vi "Voltage - Finite Output.vi"() -> ()   [LabVIEW 2011]
doc: "This example demonstrates how to generate a finite amount of data from a buffer in your computer's memory."
uses:
  <libdir>/resource/objmgr/daqmx.rc
  <vilib>/DAQmx/create/channels.llb/DAQmx Create Channel (AO-Voltage-Basic).vi
  <vilib>/DAQmx/configure/trigger.llb/DAQmx Start Trigger (Analog Edge).vi
  <vilib>/DAQmx/configure/trigger.llb/DAQmx Start Trigger (Digital Edge).vi
  <vilib>/Utility/error.llb/DialogType.ctl
  <vilib>/DAQmx/write.llb/DAQmx Write (Analog Wfm 1Chan NSamp).vi
  <vilib>/DAQmx/configure/timing.llb/DAQmx Timing (Use Waveform).vi
  <vilib>/Utility/file.llb/Read Delimited Spreadsheet (DBL).vi
panel:
  out "Samples":i32
  out "appended path":path
  in  "amplitude":dbl=1.0 format="%0.2p"
  in  "Trigger Type":T1(tab)
  in  "Edge":i32(ring)=10280 items=["Rising"=10280, "Falling"=10171]
  in  "Digital Trigger Source":tag
  in  "Level (V)":dbl format="%0.2f"
  in  "Hysteresis (V)":dbl
  in  "Slope":i32(ring)=10280 items=["Rising"=10280, "Falling"=10171]
  in  "Analog Trigger Source":string="APFI0"
  out "Waveform Graph":waveform(dbl)(graph)
  in  "Sample Rate":dbl=1000.0
  in  "Physical Channel(s)":tag="Dev1/ao0"
  out "Actual Sample Rate":dbl=1000.0 format="%0.2f"
  # "Channel Settings"
  # "Output"
  # "Timing and Buffer Settings"
  # "Trigger Settings"
  # "Waveform Settings"
  # "The number of elements in the waveform array must equal the number of channels in the task."
  # "To configure and use a start trigger you must have the necessary tab selected above.  Not all hardware supports triggering--refer to your device documentation for more info."
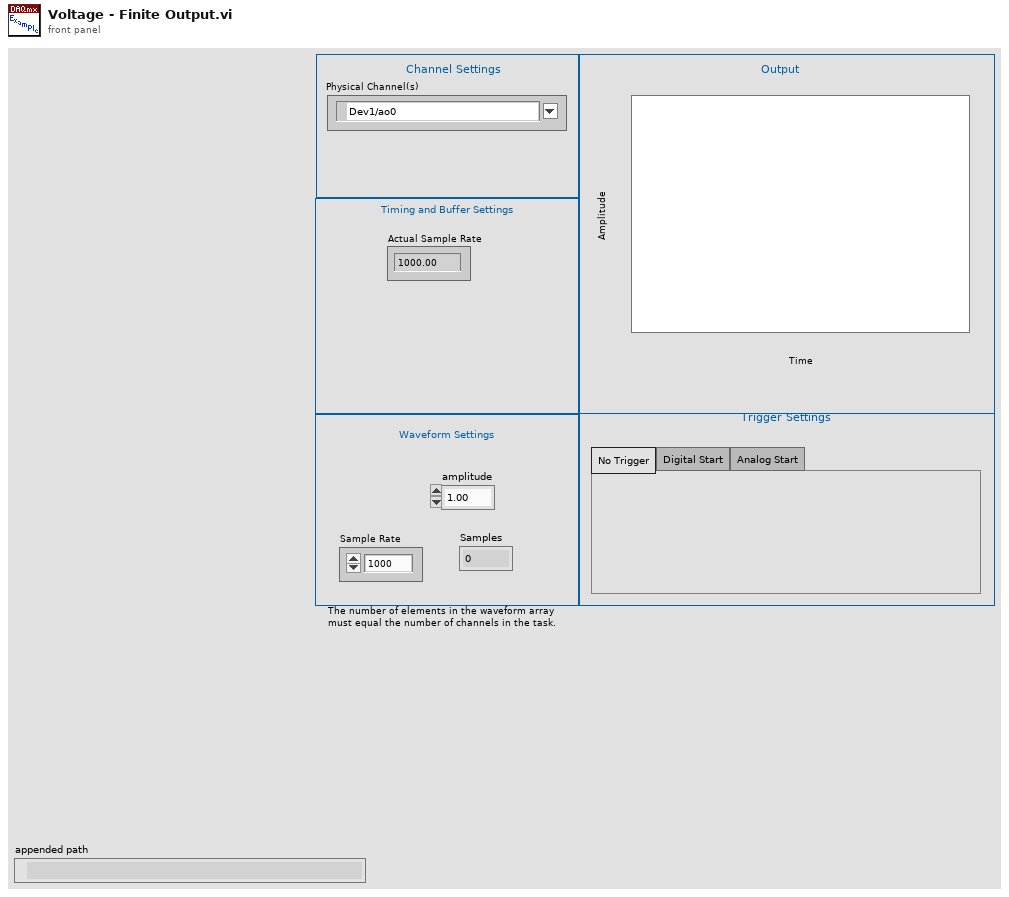
[diagram p1: front panel]
types:
  T1 = enum32{"No Trigger", "Digital Start", "Analog Start"}
  T2 = typedef "DialogType.ctl" = u16
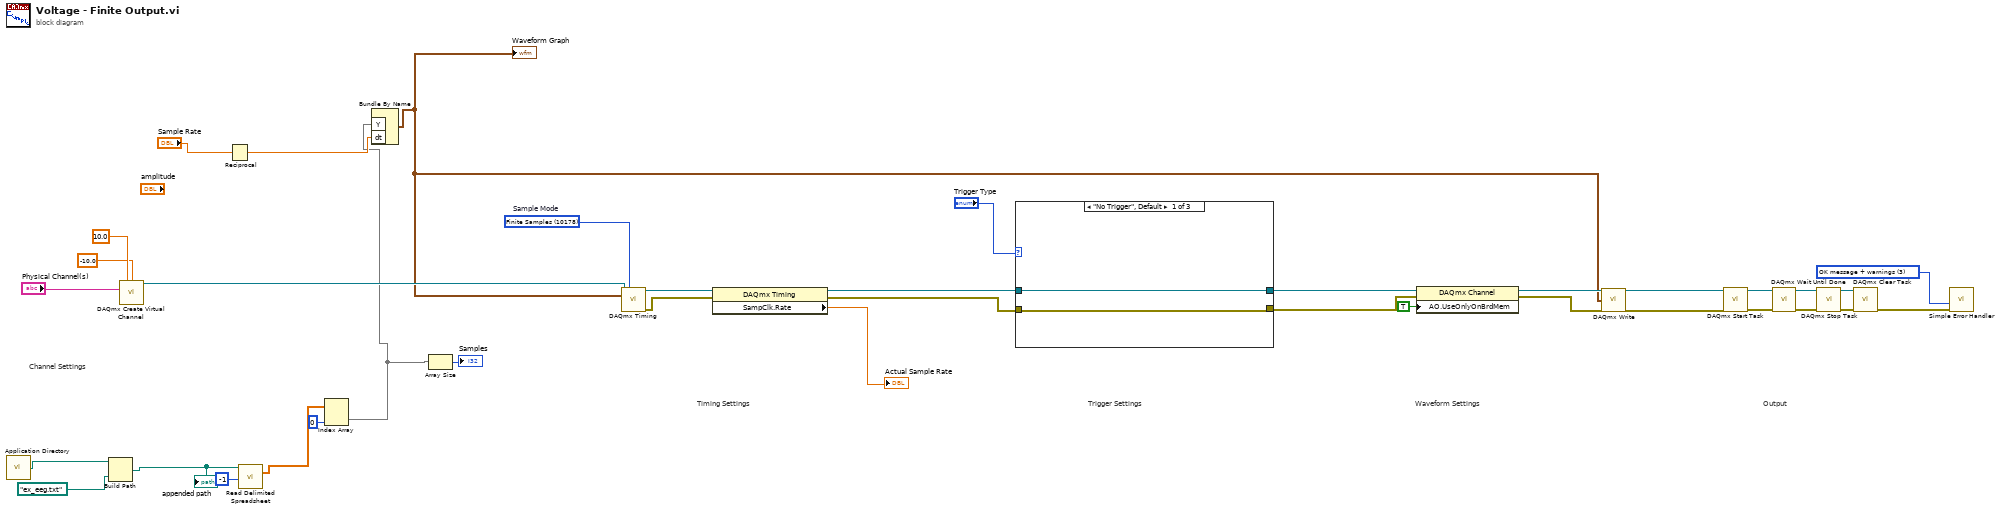
[diagram p0: block diagram]
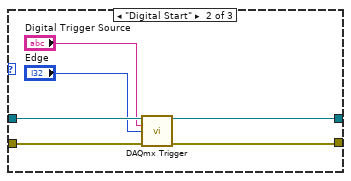
[diagram p2: hidden frame]
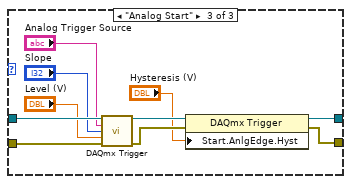
[diagram p3: hidden frame]
diagram:
  w19 = T2 3 items=["no dialog", "OK message", "continue or stop message", "OK message + warnings", "continue/stop + warnings"] ("type of dialog (OK msg:1)")
  w35 = 10178 items=["Finite Samples"=10178, "Continuous Samples"=10123, "Hardware Timed Single Point"=12522]  # Sample Mode
  # "Output"
  # "Trigger Settings"
  # "Waveform Settings"
  # "Timing Settings"
  # "Channel Settings"
  n1 = call <vilib>:"Application Directory.vi"() -> ("Application Directory"=w7:path)
  n2 = Build Path(base path=w7, name or relative path=path "ex_eeg.txt" ("file path (dialog if empty)")) -> (appended path=w8:path)
  "appended path" <- w8
  n3 = call-poly <vilib>:"DAQmx Create Virtual Channel.vi"("maximum value"=10.0, "minimum value"=-10.0, "physical channels"="Physical Channel(s)") -> ("task out"=w34:refnum<k21>)  [unwired: 11 in, 1 out]
  n4 = Reciprocal(x="Sample Rate") -> (1/x=w11:dbl)
  n5 = call-poly <vilib>:"Read Delimited Spreadsheet.vi"("file path (dialog if empty)"=w8, "number of rows (all:-1)"=-1) -> ("all rows"=w6:dbl[][])  [unwired: 8 in, 5 out]
  n6 = Index Array(array=w6, index (col)=0 ("disabled index (col)")) -> (element=w2:dbl[])  [unwired: 1 in]
  n7 = Bundle By Name("Y"=w2, "dt"=w11) -> (w13:waveform(dbl))  [unwired: 1 in]
  "Waveform Graph" <- w13
  n8 = Array Size(array=w2) -> (size(s)=→"Samples":i32)
  n9 = call-poly <vilib>:"DAQmx Timing.vi"("task/channels in"=w34, "sample mode"=w35, "waveform"=w13) -> ("task out"=w37:refnum<k21>, "error out"=w36:errorcluster)  [unwired: 11 in]
  n10 = property class="DAQmx Timing"(reference=w37, error in=w36) -> (reference out=w30:refnum<k21>, error out=w29:errorcluster, "SampClk.Rate"=→"Actual Sample Rate":dbl)
  n11 = case shown="\"No Trigger\", Default" "Trigger Type" {
    tunnel: w30 -> [w39 w45 w55]
    tunnel: w29 -> [w38 w44 w54]
    tunnel: [w39 w43 w52] -> w15
    tunnel: [w38 w42 w51] -> w17
    frame "No Trigger", Default {
    }
    frame "Digital Start" {
      n12 = call-poly <vilib>:"DAQmx Trigger.vi"("task/channels in"=w45, "source"="Digital Trigger Source", "edge"="Edge", "error in"=w44) -> ("task out"=w43:refnum<k21>, "error out"=w42:errorcluster)  [unwired: 10 in]
    }
    frame "Analog Start" {
      n13 = call-poly <vilib>:"DAQmx Trigger.vi"("task/channels in"=w55, "source"="Analog Trigger Source", "slope"="Slope", "level"="Level (V)", "error in"=w54) -> ("task out"=w50:refnum<k21>, "error out"=w49:errorcluster)  [unwired: 9 in]
      n14 = property class="DAQmx Trigger"(reference=w50, error in=w49, "Start.AnlgEdge.Hyst"="Hysteresis (V)") -> (reference out=w52:refnum<k21>, error out=w51:errorcluster)
    }
  }
  n15 = property class="DAQmx Channel"(reference=w15, error in=w17, "AO.UseOnlyOnBrdMem"=TRUE) -> (reference out=w14:refnum<k21>, error out=w16:errorcluster)
  n16 = call-poly <vilib>:"DAQmx Write.vi"("task/channels in"=w14, "data"=w13, "error in"=w16) -> ("task out"=w28:refnum<k21>, "error out"=w27:errorcluster)  [unwired: 10 in, 1 out]
  n17 = call <vilib>:"DAQmx Start Task.vi"("task/channels in"=w28, "error in"=w27) -> ("task out"=w26:refnum<k21>, "error out"=w25:errorcluster)  [unwired: 12 in]
  n18 = call <vilib>:"DAQmx Wait Until Done.vi"("task/channels in"=w26, "error in"=w25) -> ("task out"=w21:refnum<k21>, "error out"=w20:errorcluster)  [unwired: 12 in]
  n19 = call <vilib>:"DAQmx Stop Task.vi"("task/channels in"=w21, "error in"=w20) -> ("task out"=w23:refnum<k21>, "error out"=w22:errorcluster)  [unwired: 12 in]
  n20 = call <vilib>:"DAQmx Clear Task.vi"("task in"=w23, "error in"=w22) -> ("error out"=w33:errorcluster)  [unwired: 13 in]
  n21 = call <vilib>:"Simple Error Handler.vi"("type of dialog (OK msg:1)"=w19, "error in (no error)"=w33) -> ()  [unwired: 3 in, 5 out]
